vi "Get Class Parents.vi"(10 "LVClassLibrary in":refnum<vi>) -> (2 "Array":refnum<vi>[](array[refnum]), 4 "Array 6":string[](array[string]))   [LabVIEW 2018, in "ORM Scripter.lvclass"]
uses:
  ORM Scripter.lvclass
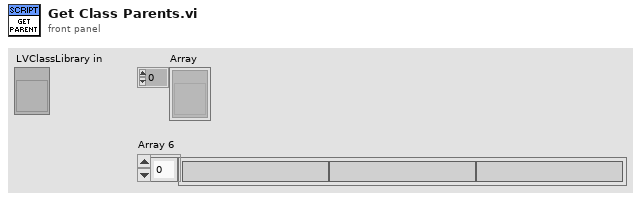
[diagram p1: front panel]
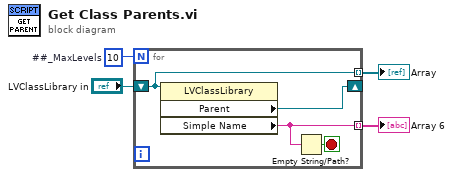
[diagram p0: block diagram]
diagram:
  w4 = 10  # ##_MaxLevels
  n1 = for {
    N: w4 -> [_]
    shift-right: [w8] -> _
    shift-left: "LVClassLibrary in" -> [w7]
    tunnel: [w6] -> w1 mode=indexing
    tunnel: [w7] -> w2 mode=indexing
    stop <- w5 stop-if-true
    n2 = property class="LVClassLibrary"(reference=w7) -> ("Parent"=w8:refnum<vi>, "Simple Name"=w6:string)  [unwired: 1 in, 2 out]
    n3 = Empty String/Path?(string/path=w6) -> (empty?=w5:bool)
  }
  "Array 6" <- w1
  "Array" <- w2
